vi "Query Port level.vi"(8 "error in (no error)":errorcluster, 10 "i (1)":T1=enum."PORT 1", 11 "VISA resource name":refnum<visa-resource-name>) -> (0 "error out":errorcluster, 2 "output":dbl, 3 "VISA resource name out":refnum<visa-resource-name>)   [LabVIEW 2009, in "SR400.lvlib"]
doc: "PL i { ,v }\nThe PL command sets and reads thePORT1 and\nPORT2 output levels. i=1 or 2 to select PORT1 or\nPORT 2 and is required. If v is included, the\noutput level is set to v Volts where -10.000 <= v\n<= 10.000. The resolution is 0.005 V (5 mV). If v\nis absent, the output level is returned. If the Port\noutput mode is SCAN, the PL command sets and\nreads the starting value of the level. Changing the\nlevel during a scan will cause the level to be set to\nthe new value on the next count period. Note that\nthe scan is not reset. Reading the level during a\nscan always returns the starting value, not the\ncurrent value."
uses:
  SR400.lvlib
  Typedefs.llb/PORT Output.ctl
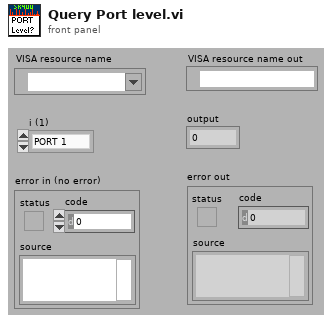
[diagram p1: front panel]
types:
  T1 = typedef "SR400.lvlib/PORT Output.ctl" = enum16{"(not used)", "PORT 1", "PORT 2"}
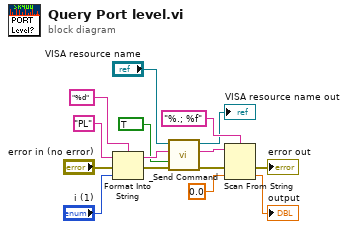
[diagram p0: block diagram]
diagram:
  n1 = Format Into String(format string="%d", initial string="PL" ("command"), error in="error in (no error)", "i (1)") -> (resulting string=w6:string, error out=w5:errorcluster)
  n2 = call "_Send Command.vi"("error in (no error)"=w5, "Query? (F)"=TRUE, "Command"=w6, "VISA resource name"="VISA resource name") -> ("error out"=w2:errorcluster, "Response"=w3:string, "VISA resource name out"=→"VISA resource name out":refnum<visa-resource-name>)  [unwired: 5 out]
  n3 = Scan From String(format string="%.; %f", input string=w3, error in=w2, default 1=0.0 ("default value 1")) -> (error out=→"error out":errorcluster, output 1=→"output":dbl)  [unwired: 1 in, 2 out]
